vi "Begin.vi"(8 "error in (no error)":errorcluster, 10 "variant in":variant, 11 "Old Drive Robot in":refnum<class "Outlaw.lvclass">) -> (0 "error out":errorcluster, 3 "Old Drive Robot out":refnum<class "Outlaw.lvclass">)   [LabVIEW 2019, in "Robot.lvlib" / "Outlaw.lvclass"]
uses:
  Outlaw.lvclass
  Robot.lvclass
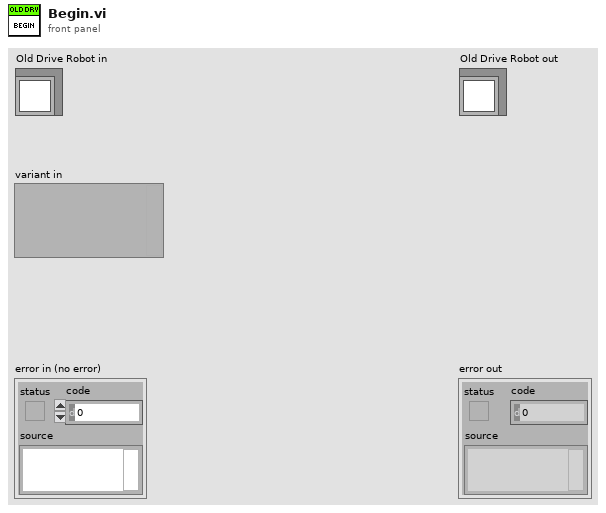
[diagram p1: front panel]
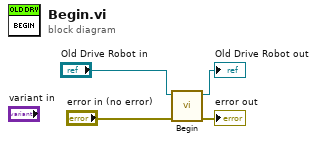
[diagram p0: block diagram]
diagram:
  n1 = call-parent "Begin.vi"("error in (no error)"="error in (no error)", "Robot in"="Old Drive Robot in") -> ("error out"=→"error out":errorcluster, "Robot out"=→"Old Drive Robot out":refnum<class "Outlaw.lvclass">)  [unwired: 8 in]
